vi "Handle to Pointer.vi"(4 "error in (no error)":errorcluster, 7 "Handle":i32) -> (0 "error out":errorcluster, 2 "Pointer":i32, 3 "Duplicate Handle":i32)   [LabVIEW 2011]
doc: "Use this VIs to get a Pointer from a Handle value."
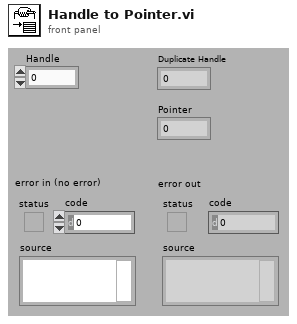
[diagram p1: front panel]
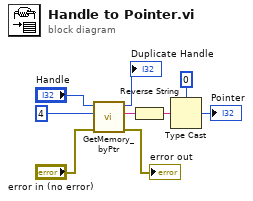
[diagram p0: block diagram]
diagram:
  n1 = call "GetMemory_byPtr.vi"("error in (no error)"="error in (no error)", "Data Size(1)"=4 ("Data Size"), "Pointer"="Handle") -> ("error out"=→"error out":errorcluster, "data"=w7:string, "Duplicate Pointer"=→"Duplicate Handle":i32)  [unwired: 3 out]
  n2 = Reverse String(1:w7) -> (0:w6:string)
  n3 = Type Cast(type=0 ("Data Size"), x=w6) -> (*(type *) &x=→"Pointer":i32)
